vi "NS_WriteAttribute.vi"(0 "object in":refnum<class "NativeSubTemplate_4x4x4.lvclass">, 5 "error in (no error)":errorcluster) -> (14 "object out":refnum<class "NativeSubTemplate_4x4x4.lvclass">, 19 "error out":errorcluster)   [LabVIEW 2014, in "NativeSubTemplate_4x4x4.lvclass"]
uses:
  <resource>/Framework/Providers/Open_GDS/ClassProviders/Provider_LvNativeClass/Templates/NativeSubTemplate_4x4x4/NativeSubTemplate_4x4x4.lvclass
  <resource>/Framework/Providers/Open_GDS/ClassProviders/Provider_LvNativeClass/Templates/NativeSubTemplate_4x4x4/NativeSubTemplate_4x4x4.lvclass/NativeSubTemplate_4x4x4.ctl
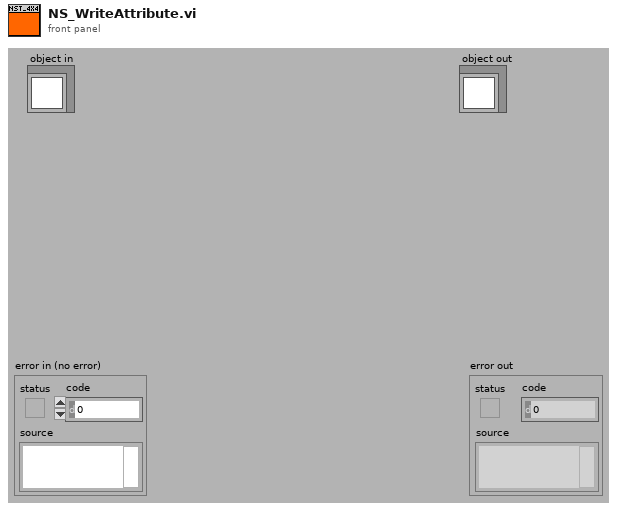
[diagram p1: front panel]
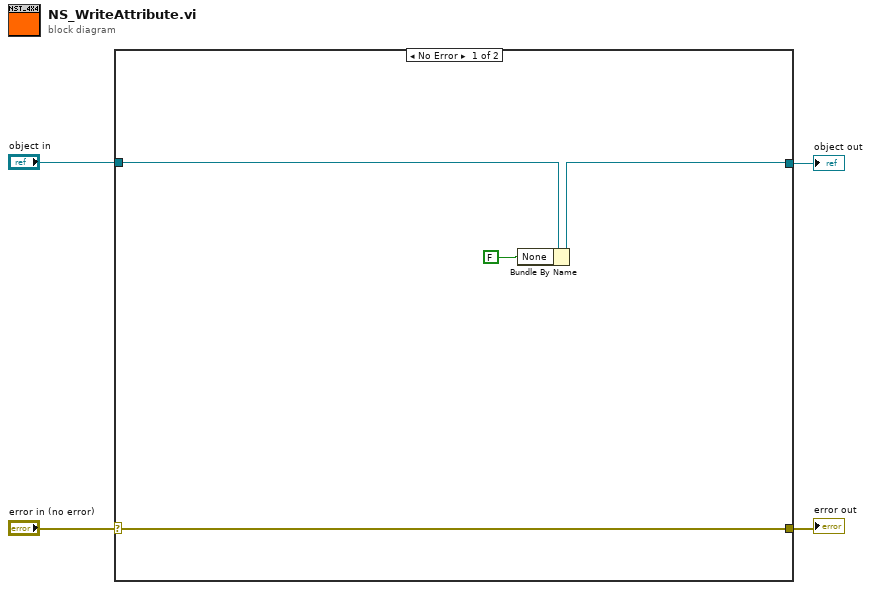
[diagram p0: block diagram]
diagram:
  n1 = case shown="No Error" "error in (no error)" {
    selector: "error in (no error)" -> [w8 w10]
    tunnel: [w8 w10] -> w3
    tunnel: [w6 w9] -> w1
    tunnel: "object in" -> [w7 w9]
    frame No Error {
      n2 = Bundle By Name(cluster=w7, "None"=FALSE) -> (w6:refnum<class "NativeSubTemplate_4x4x4.lvclass">)
    }
    frame Error {
    }
  }
  "error out" <- w3
  "object out" <- w1
